vi "UV_LED switch.vi"(6 "ForceOff":bool=TRUE, 7 "On/Off (F:off)":bool, 8 "error in":errorcluster, 10 "CHN":T1=255 items=["All"=255, "CH1"=1, "CH2"=2, "CH3"=3, "CH4"=4], 11 "VISA resource":refnum<visa-resource-name>="COM5") -> (0 "error out":errorcluster, 2 "CH_change":u8, 3 "VISA resource out":refnum<visa-resource-name>, 5 "Err?":bool)   [LabVIEW 2014]
uses:
  TypeDef/UVLed_func.ctl
  TypeDef/UVLed_channel.ctl
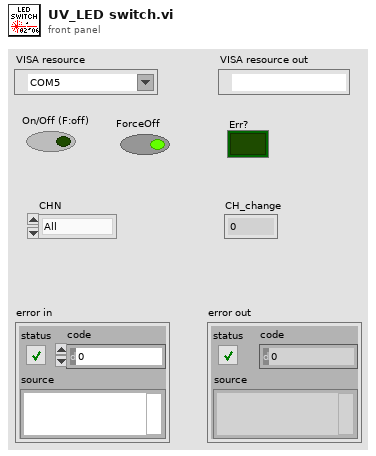
[diagram p1: front panel]
types:
  T1 = typedef "UVLed_channel.ctl" = u16
  T2 = typedef "UVLed_func.ctl" = u16
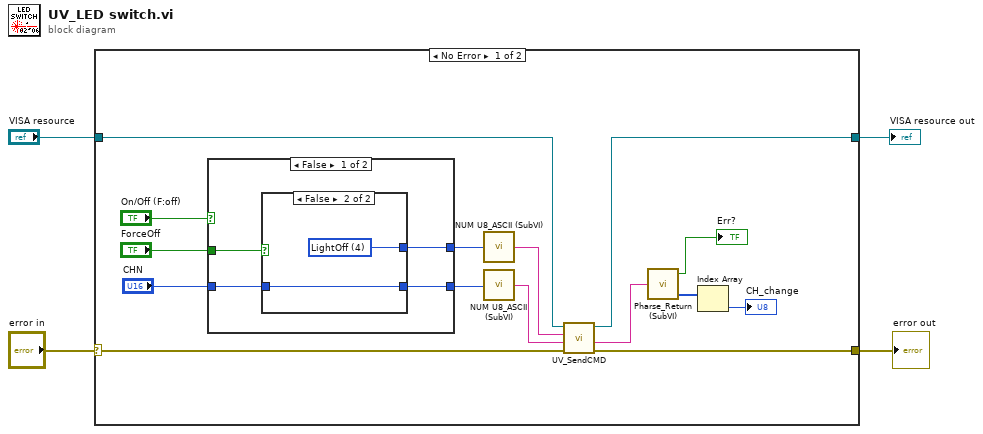
[diagram p0: block diagram]
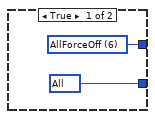
[diagram p2: hidden frame]
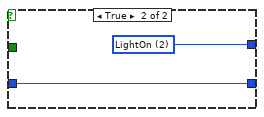
[diagram p3: hidden frame]
diagram:
  n1 = case shown="No Error" "error in" {
    selector: "error in" -> [w16 w31]
    tunnel: [w14 w31] -> w3
    tunnel: "VISA resource" -> [w17 w30]
    tunnel: [w12 w30] -> w1
    frame No Error {
      n2 = case shown="False" "On/Off (F:off)" {
        tunnel: [w23 w29] -> w19
        tunnel: "CHN" -> [w20 w28]
        tunnel: [w21 w28] -> w10
        tunnel: "ForceOff" -> [w22 _]
        frame False {
          n3 = case shown="False" w22 {
            tunnel: [w25 w27] -> w23
            tunnel: [w24 w26] -> w21
            tunnel: w20 -> [_ w26]
            frame True {
              w24 = T1 255 items=["All"=255, "CH1"=1, "CH2"=2, "CH3"=3, "CH4"=4] ("CHN")
              w25 = T2 6 items=["GetAllStatus"=0, "LightOn"=2, "LightOff"=4, "AllForceOff"=6, "GetMenuChnPara"=10, "SetMenuChnPara"=12, "GetAutoChnPara"=14, "SetAutoChnPara"=16, "GetMenuTemplate"=18, "SetMenuTemplate"=20, "GetAutoTemplate"=22, "SetAutoTemplate"=24, "GetTemplatePara"=26, "SetTemplatePara"=28, "GetMode"=30, "SetMode"=32, "ChkErr"=240] ("Function")
            }
            frame False {
              w27 = T2 4 items=["GetAllStatus"=0, "LightOn"=2, "LightOff"=4, "AllForceOff"=6, "GetMenuChnPara"=10, "SetMenuChnPara"=12, "GetAutoChnPara"=14, "SetAutoChnPara"=16, "GetMenuTemplate"=18, "SetMenuTemplate"=20, "GetAutoTemplate"=22, "SetAutoTemplate"=24, "GetTemplatePara"=26, "SetTemplatePara"=28, "GetMode"=30, "SetMode"=32, "ChkErr"=240] ("Function")
            }
          }
        }
        frame True {
          w29 = T2 2 items=["GetAllStatus"=0, "LightOn"=2, "LightOff"=4, "AllForceOff"=6, "GetMenuChnPara"=10, "SetMenuChnPara"=12, "GetAutoChnPara"=14, "SetAutoChnPara"=16, "GetMenuTemplate"=18, "SetMenuTemplate"=20, "GetAutoTemplate"=22, "SetAutoTemplate"=24, "GetTemplatePara"=26, "SetTemplatePara"=28, "GetMode"=30, "SetMode"=32, "ChkErr"=240] ("Function")
        }
      }
      n4 = call "NUM U8_ASCII (SubVI).vi"("Numeric"=w19) -> ("String out"=w18:string)
      n5 = call "NUM U8_ASCII (SubVI).vi"("Numeric"=w10) -> ("String out"=w15:string)
      n6 = call "UV_SendCMD.vi"("error in"=w16, "value"=w15, "function"=w18, "VISA resource name"=w17) -> ("error out"=w14:errorcluster, "response"=w13:string, "VISA resource name out"=w12:refnum<visa-resource-name>)  [unwired: 5 in]
      n7 = call "Pharse_Return (SubVI).vi"("buffer in"=w13) -> ("byte array"=w6:u8[], "Err?"=→"Err?":bool)  [unwired: 2 in, 1 out]
      n8 = Index Array(array=w6) -> (element=→"CH_change":u8)  [unwired: 1 in]
    }
    frame Error {
    }
  }
  "error out" <- w3
  "VISA resource out" <- w1
